vi "XML Build Poll Request Frame.vi"(2 "XML-Message":string, 9 "error in (no error)":errorcluster caption="Fehler (Eingang, kein Fehler)") -> (0 "XML-Message fertig":string, 6 "error out":errorcluster caption="Fehler (Ausgang)")   [LabVIEW 2020, in "FT-IR.lvlib" / "TOOLweb Interface.lvlib" / "TOOLweb Interface Hilfs-VIs.lvlib"]
doc: "Gibt allen Poll-Request-Zeilen, die in \"XML-Message\" gemeinsam übegeben werden, mit dem Start-Tag <PollRequest> und dem End-Tag </PollRequest> den Rahmen für eine einzige und damit schnelle XML-Poll-Request Anfrage.\n\nDer Ausgangs-String \"XML-Message fertig\" kann mit dem VI \"http XML send receive\" gesendet werden."
uses:
  TOOLweb Interface Hilfs-VIs.lvlib
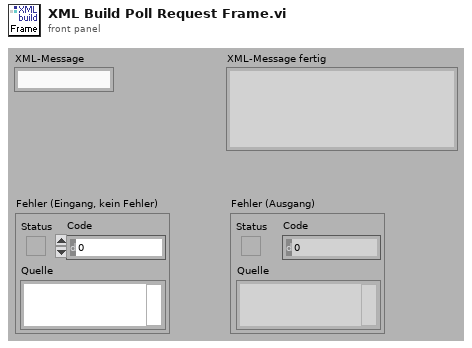
[diagram p1: front panel]
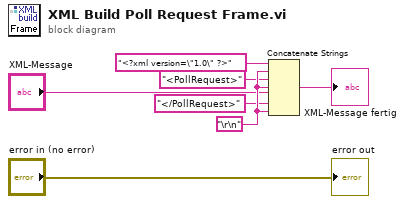
[diagram p0: block diagram]
diagram:
  w6 = "\r\n"
  n1 = Concatenate Strings("<?xml version=\"1.0\" ?>" ("Daten (Eingang)"), w6, "<PollRequest>" ("Daten (Eingang)"), w6, "XML-Message", "</PollRequest>" ("Daten (Eingang)"), w6) -> (→"XML-Message fertig":string)
  "error out" <- "error in (no error)"
